vi "Write Connection ID.vi"(10 "connection ID":refnum<k5>, 11 "TCP Stream in":refnum<class "TCP Stream.lvclass">) -> (3 "TCP Stream out":refnum<class "TCP Stream.lvclass">)   [LabVIEW 2020, in "TCP Stream.lvclass"]
uses:
  TCP Stream.lvclass
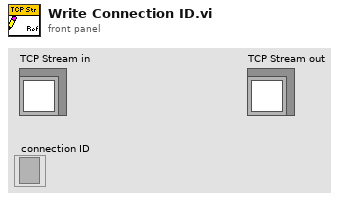
[diagram p1: front panel]
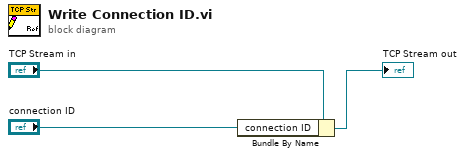
[diagram p0: block diagram]
diagram:
  n1 = Bundle By Name(cluster="TCP Stream in", "connection ID"="connection ID") -> (→"TCP Stream out":refnum<class "TCP Stream.lvclass">)
